vi "demo_xtable.vi"() -> ()   [LabVIEW 2016]
uses:
  XControl 1.xctl
  ZebraTable.lvlibp/XControl 1.xctl
panel:
  out "ALL vi":string[][](table)
  in  "XControl 2":string[][](xcontrol)
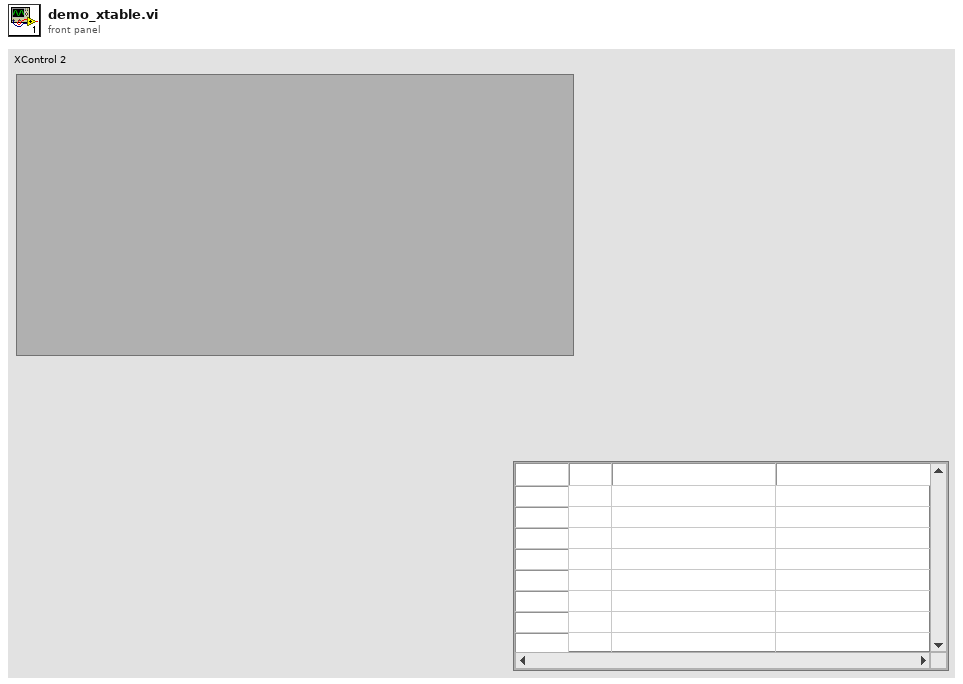
[diagram p1: front panel]
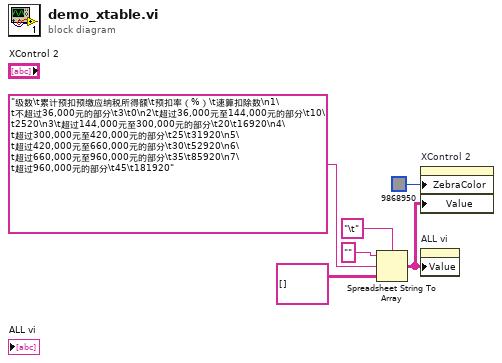
[diagram p0: block diagram]
diagram:
  n1 = Spreadsheet String To Array(delimiter (Tab)="\t", format string="", spreadsheet string="级数\t累计预扣预缴应纳税所得额\t预扣率（%）\t速算扣除数\n1\t不超过36,000元的部分\t3\t0\n2\t超过36,000元至144,000元的部分\t10\t2520\n3\t超过144,000元至300,000元的部分\t20\t16920\n4\t超过300,000元至420,000元的部分\t25\t31920\n5\t超过420,000元至660,000元的部分\t30\t52920\n6\t超过660,000元至960,000元的部分\t35\t85920\n7\t超过960,000元的部分\t45\t181920", array type (2D Dbl)=string[][] [] ("XControl 1")) -> (array=w1:string[][])
  n2 = property on="XControl 2" class="XControl 1 (strict)"("ZebraColor"=u32 9868950, "Value"=w1) -> ()  [unwired: 2 in, 2 out]
  n3 = property on="ALL vi" class="Tbl (strict)"("Value"=w1) -> ()  [unwired: 2 in, 2 out]
